vi "ConditioningState-Case.vi"() -> ()   [LabVIEW 2014]
uses:
  ParamsArray.ctl
  Licker.lvclass
  Juicer.lvclass
  Acquisition.lvclass
  Stimulus.lvclass
  state.lvsc/Outputs.ctl
  state.lvsc/Inputs.ctl
  <vilib>/Utility/file.llb/Read From Spreadsheet File (DBL).vi
  state.lvsc
panel:
  out "Waveform Chart":dbl(graph)
  out "size(s) 4":i32
  out "size(s) 3":i32
  out "size(s) 2":i32
  out "size(s)":i32
  out "error out 2":errorcluster
  out "x-y":dbl
  out "Active States":string[](array[string])
  in  "screen_setup":u16(ring) items=["Default", "1"]
  out "queue#":i32
  in  "Probes":enum16{"Testing", "1-5", "6-10"}(ring)=enum."6-10"
  in  "Display":bool
  out "Mon params":dbl[][](array[numeric])=[[100.0, 100.0, 0.0, 0.0], [100.0, 100.0, 100.0, 0.0], [100.0, 100.0, 200.0, 0.0], [100.0, 100.0, 300.0, 0.0], [100.0, 100.0, 400.0, 0.0]]
  out "Air":bool[](array[boolean])
  out "Optical traces":waveform(dbl)[](graph)
  out "CS":bool[](array[boolean])
  out "Number of Licks":dbl[](array[numeric]) caption="#Licks"
  in  "LICK":bool[](array[boolean])=[FALSE, FALSE, FALSE, FALSE, FALSE]
  out "Elapsed Time":dbl[](array[numeric]) caption="Time to Stim"
  out "Rewards Given":dbl[](array[numeric]) caption="#Rew"
  in  "Thr":dbl[](array[numeric])=[10.0, 10.0, 10.0, 10.0, 10.0]
  out "Water":bool[](array[boolean])
  out "Licks":bool[](array[boolean])
  out "error out":errorcluster
  out "Sti":i32
  in  "RUN":bool[](array[boolean])=[FALSE, FALSE, FALSE, FALSE, FALSE]
  out "Lick":i32
  out "Acq":i32
  out "Jui":i32
  in  "REC":bool[](array[boolean])=[FALSE, FALSE, FALSE, FALSE, FALSE]
  in  "Stop":bool
  in  "Params":T1={"Mice ID"=[], "ExpType"=[], "Trial Interval"=[], "Pulse Duration"=[158.0, 152.0, 156.0, 167.0, 172.0], "microL_per_pulse"=[6.0, 6.0, 6.0, 6.0, 6.0], "Response Interval"=[1000.0, 1000.0, 1000.0, 1000.0, 1000.0], "Bad Delay"=[], "Response Period"=[], "liquid_type"="water", "Stimuli"=[], "Rewarded Stimuli"=[], "Air Dur"=400.0} {"Air Dur" format="%#_13g"}
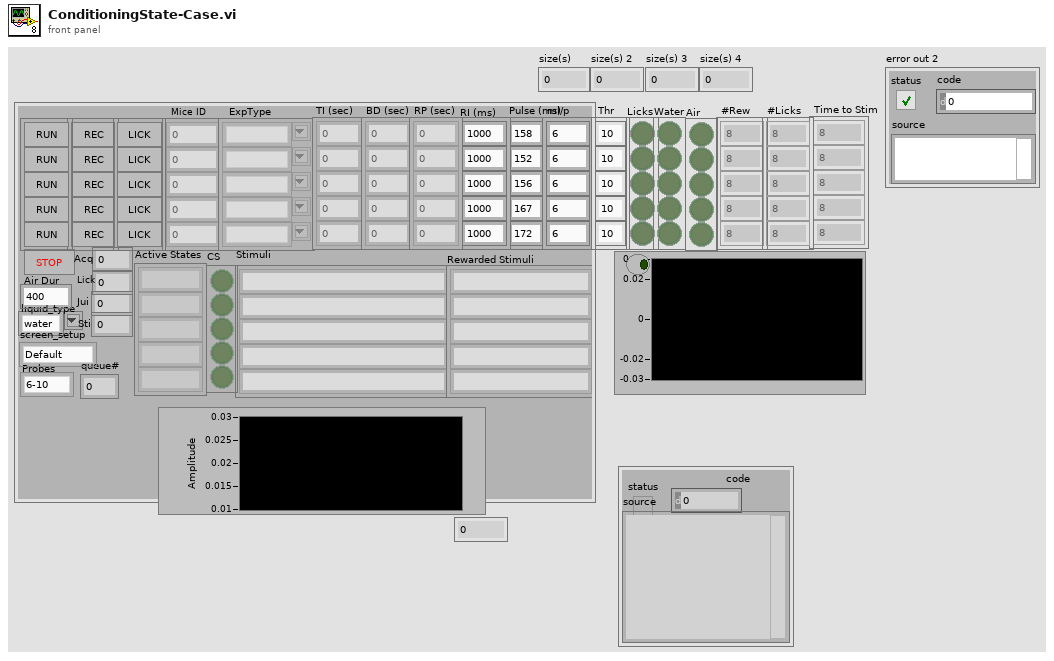
[diagram p1: front panel]
types:
  T1 = typedef "ParamsArray.ctl" = cluster{"Mice ID":dbl[], "ExpType":string[], "Trial Interval":dbl[], "Pulse Duration":dbl[], "microL_per_pulse":dbl[], "Response Interval":dbl[], "Bad Delay":dbl[], "Response Period":dbl[], "liquid_type":string, "Stimuli":string[], "Rewarded Stimuli":string[], "Air Dur":dbl}
  T2 = typedef "state.lvsc/Outputs.ctl" = cluster{"Stimulus.lvclass":refnum<class "Stimulus.lvclass">, "error out":errorcluster, "State":string, "Index":dbl, "Correct Response":bool}
  T3 = enum16{"air_delivery", "beh_session", "stim_periods", "licks", "liquid_delivery", ""}
  T4 = enum16{"Get Time", "Get Elapsed Time", "Reset Elapsed Time"}
  T5 = typedef "state.lvsc/Inputs.ctl" = cluster{"Acquisition.lvclass":refnum<class "Acquisition.lvclass">, "Stimulus.lvclass":refnum<class "Stimulus.lvclass">, "Juicer.lvclass":refnum<class "Juicer.lvclass">, "Index":dbl, "error in (no error)":errorcluster, "Lick":bool, "State":string}
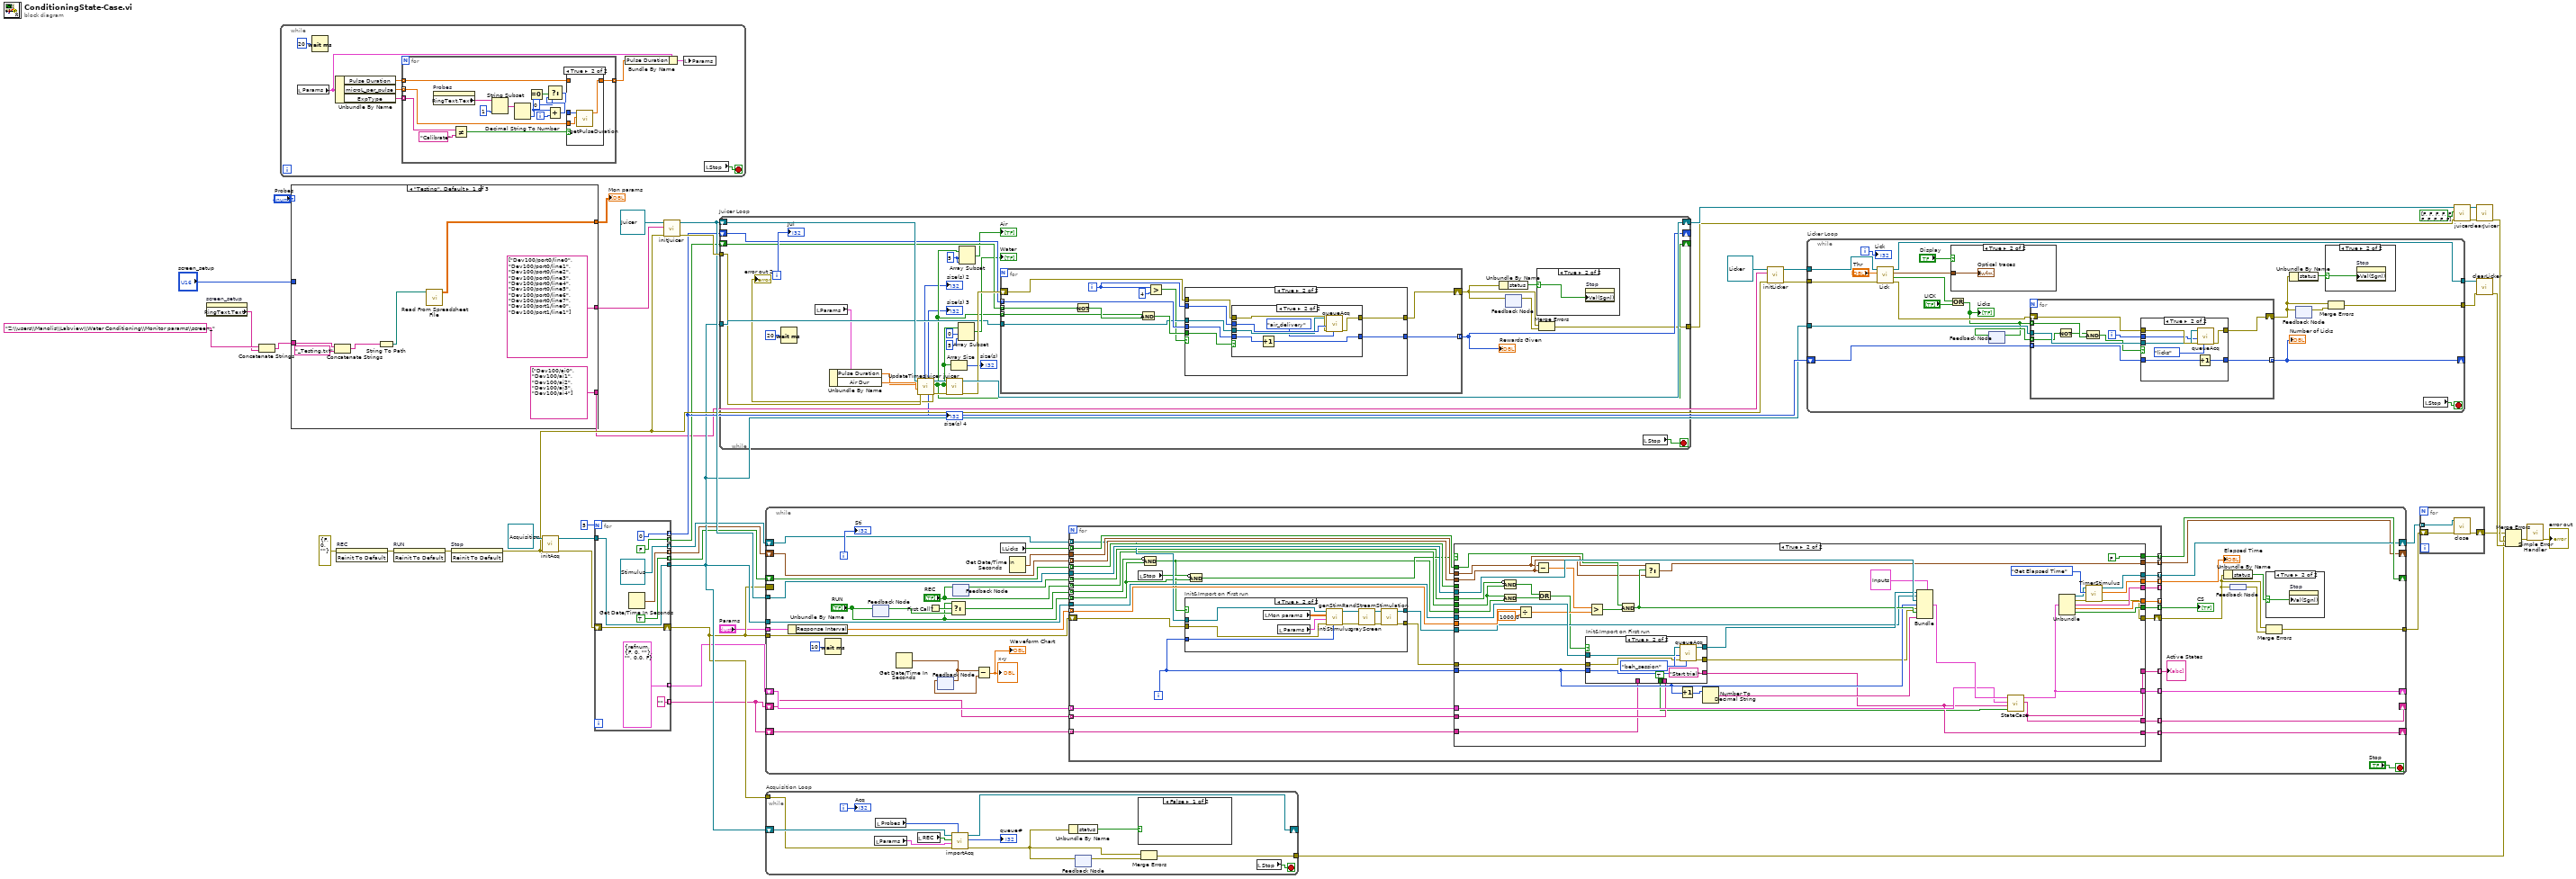
[diagram p0: block diagram]
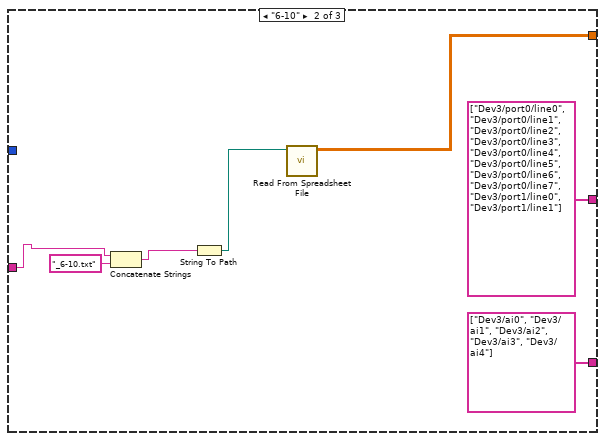
[diagram p3: hidden frame]
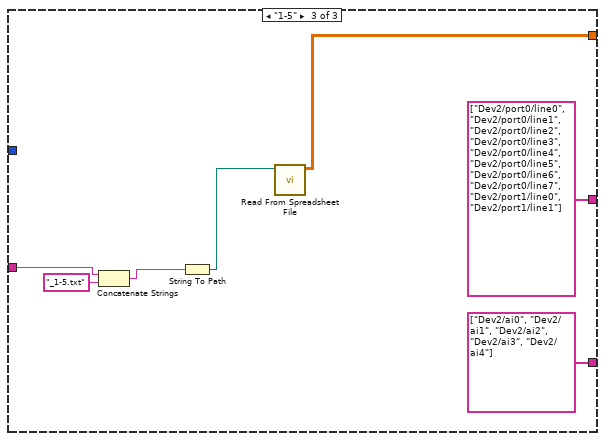
[diagram p4: hidden frame]
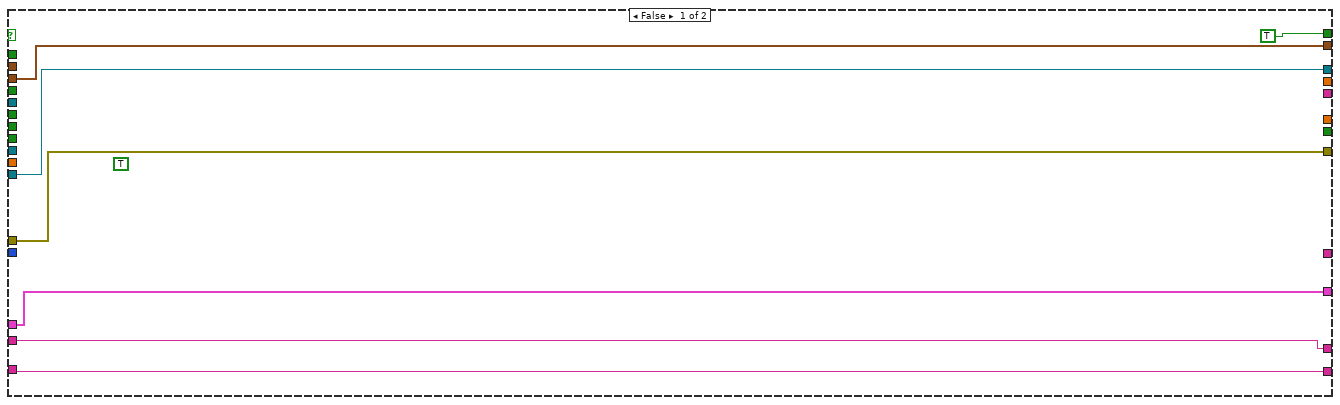
[diagram p7: hidden frame]
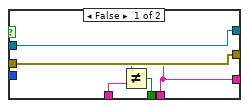
[diagram p8: hidden frame]
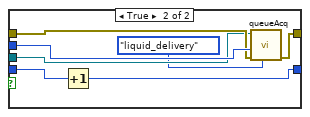
[diagram p14: hidden frame]
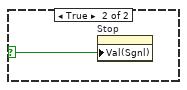
[diagram p16: hidden frame]
diagram:
  n1 = property on="screen_setup" class="Ring (strict)"() -> ("RingText.Text"=w4:string)  [unwired: 2 in, 2 out]
  n2 = Concatenate Strings("Z:\\users\\Manolis\\Labview\\Water Conditioning\\Monitor params\\screen_" ("file path (dialog if empty)"), w4) -> (w3:string)
  n3 = while {
    stop <- w55 stop-if-true
    n4 = local read "Params"() -> (w49:T1)
    n5 = Wait (ms)(milliseconds to wait=u32 20) -> ()  [unwired: 1 out]
    n6 = Unbundle By Name(w49) -> ("Pulse Duration"=w51:dbl[], "microL_per_pulse"=w53:dbl[], "ExpType"=w48:string[])
    n7 = for {
      tunnel: w53 -> [w66] mode=indexing
      tunnel: [w64] -> w52 mode=indexing
      tunnel: w51 -> [w63] mode=indexing
      tunnel: w48 -> [w62] mode=indexing
      i -> [w70]
      n8 = property on="Probes" class="Enum (strict)"() -> ("RingText.Text"=w67:string)  [unwired: 2 in, 2 out]
      n9 = Not Equal?(x=w62, y="Calibrate") -> (x != y?=w61:bool)
      n10 = String Subset(string=w67, length (rest)=1 ("length (rest)")) -> (substring=w69:string)  [unwired: 1 in]
      n11 = Decimal String To Number(string=w69) -> (number=w58:i32)  [unwired: 2 in, 1 out]
      n12 = Equal To 0?(x=w58) -> (x = 0?=w57:bool)
      n13 = Add(x=w58, y=w70) -> (x+y=w60:i32)
      n14 = Select(t=0, s=w57, f=w60) -> (s? t:f=w59:i32)
      n15 = case shown="True" w61 {
        tunnel: w59 -> [_ w74]
        tunnel: w66 -> [_ w73]
        tunnel: [w71 w72] -> w64
        tunnel: w63 -> [w71 _]
        frame False {
        }
        frame True {
          n16 = call "getPulseDuration.vi"("target microL/pulse"=w73, "Probe #"=w74) -> ("Pulse Duration"=w72:dbl)  [unwired: 9 in]
        }
      }
    }
    n17 = Bundle By Name(cluster=w49, "Pulse Duration"=w52) -> (w50:T1)
    n18 = local write "Params"(w50) -> ()
    n19 = local read "Stop"() -> (w55:bool)
  }
  n20 = case shown="\"Testing\", Default" "Probes" {
    tunnel: [w75 w82 w89] -> w16
    tunnel: [string[] ["Dev100/port0/line0", "Dev100/port0/line1", "Dev100/port0/line2", "Dev100/port0/line3", "Dev100/port0/line4", "Dev100/port0/line5", "Dev100/port0/line6", "Dev100/port0/line7", "Dev100/port1/line0", "Dev100/port1/line1"] ("Lines") string[] ["Dev3/port0/line0", "Dev3/port0/line1", "Dev3/port0/line2", "Dev3/port0/line3", "Dev3/port0/line4", "Dev3/port0/line5", "Dev3/port0/line6", "Dev3/port0/line7", "Dev3/port1/line0", "Dev3/port1/line1"] ("Lines") string[] ["Dev2/port0/line0", "Dev2/port0/line1", "Dev2/port0/line2", "Dev2/port0/line3", "Dev2/port0/line4", "Dev2/port0/line5", "Dev2/port0/line6", "Dev2/port0/line7", "Dev2/port1/line0", "Dev2/port1/line1"] ("Lines")] -> w15
    tunnel: [string[] ["Dev100/ai0", "Dev100/ai1", "Dev100/ai2", "Dev100/ai3", "Dev100/ai4"] ("Lines") string[] ["Dev3/ai0", "Dev3/ai1", "Dev3/ai2", "Dev3/ai3", "Dev3/ai4"] ("Lines") string[] ["Dev2/ai0", "Dev2/ai1", "Dev2/ai2", "Dev2/ai3", "Dev2/ai4"] ("Lines")] -> w14
    tunnel: "screen_setup" -> [_ _ _]
    tunnel: w3 -> [w77 w83 w90]
    frame "Testing", Default {
      n21 = Concatenate Strings(w77, "_Testing.txt" ("string")) -> (w78:string)
      n22 = String To Path(string=w78) -> (path=w79:path)
      n23 = call-poly <vilib>:"Read From Spreadsheet File.vi"("file path (dialog if empty)"=w79) -> ("all rows"=w75:dbl[][])  [unwired: 6 in, 4 out]
    }
    frame "6-10" {
      n24 = Concatenate Strings(w83, "_6-10.txt" ("string")) -> (w85:string)
      n25 = String To Path(string=w85) -> (path=w86:path)
      n26 = call-poly <vilib>:"Read From Spreadsheet File.vi"("file path (dialog if empty)"=w86) -> ("all rows"=w82:dbl[][])  [unwired: 6 in, 4 out]
    }
    frame "1-5" {
      n27 = Concatenate Strings(w90, "_1-5.txt" ("string")) -> (w92:string)
      n28 = String To Path(string=w92) -> (path=w93:path)
      n29 = call-poly <vilib>:"Read From Spreadsheet File.vi"("file path (dialog if empty)"=w93) -> ("all rows"=w89:dbl[][])  [unwired: 6 in, 4 out]
    }
  }
  "Mon params" <- w16
  n30 = invoke on="REC" class="Arr (strict)" method="Reinit To Default"(error in=errorcluster {"status"=FALSE, "code"=0, "source"=""} ("error in (no error)")) -> (error out=w33:errorcluster)  [unwired: 2 in, 2 out]
  n31 = invoke on="RUN" class="Arr (strict)" method="Reinit To Default"(error in=w33) -> (error out=w32:errorcluster)  [unwired: 2 in, 2 out]
  n32 = invoke on="Stop" class="Bool (strict)" method="Reinit To Default"(error in=w32) -> (error out=w29:errorcluster)  [unwired: 2 in, 2 out]
  n33 = call-dynamic "initAcq.vi"("error in (no error)"=w29, "Acquisition in"=refnum<class "Acquisition.lvclass"> refnum ("Acquisition.lvclass")) -> ("error out"=w18:errorcluster, "Acquisition out"=w19:refnum<class "Acquisition.lvclass">)  [unwired: 8 in]
  n34 = for {
    N: 5 -> [_]
    tunnel: [refnum<class "Stimulus.lvclass"> refnum ("Stimulus.lvclass")] -> w30 mode=indexing
    shift-right: [w98] -> w23
    shift-left: w18 -> [w98]
    tunnel: [TRUE] -> w22 mode=indexing
    tunnel: [FALSE] -> w21 mode=indexing
    tunnel: [0] -> w25 mode=indexing
    tunnel: [w101] -> w12 mode=indexing
    tunnel: w19 -> [w100]
    tunnel: [w100] -> w24
    tunnel: [T2 {"Stimulus.lvclass"=refnum, "error out"={"status"=FALSE, "code"=0, "source"=""}, "State"="", "Index"=0.0, "Correct Response"=FALSE} ("OutputsOut")] -> w2 mode=indexing
    tunnel: ["" ("StateOut")] -> w1 mode=indexing
    n35 = Get Date/Time In Seconds() -> (seconds since 1Jan1904=w101:timestamp)
  }
  n36 = call-dynamic "initJuicer.vi"("error in (no error)"=w29, "Lines"=w15, "Juicer in"=refnum<class "Juicer.lvclass"> refnum ("Juicer.lvclass")) -> ("error out"=w44:errorcluster, "Juicer out"=w35:refnum<class "Juicer.lvclass">)  [unwired: 7 in]
  n37 = while "Juicer Loop" {
    tunnel: [w116] -> w10
    tunnel: w44 -> [w117]
    shift-right: [w131] -> w11
    shift-left: w35 -> [w132]
    shift-right: [w125] -> _
    shift-left: w25 -> [w126]
    shift-right: [w109] -> _
    shift-left: w21 -> [w124]
    tunnel: w24 -> [w118]
    i -> [w128]
    stop <- w134 stop-if-true
    w120 = 5 ("index")
    n38 = Wait (ms)(milliseconds to wait=u32 20) -> ()  [unwired: 1 out]
    n39 = local read "Params"() -> (w112:T1)
    n40 = Unbundle By Name(w112) -> ("Pulse Duration"=w111:dbl[], "Air Dur"=w113:dbl)
    n41 = call-dynamic "UpdateTimesJuicer.vi"("error in (no error)"=w117, "Air Duration"=w113, "Pulse Duration"=w111, "Juicer in"=w132) -> ("error out"=w110:errorcluster, "Juice"=w109:bool[], "Juicer out"=w133:refnum<class "Juicer.lvclass">, "size(s) 3"=→"size(s) 4":i32, "size(s) 2"=→"size(s) 3":i32, "size(s)"=→"size(s) 2":i32)  [unwired: 2 in]
    "error out 2" <- w110
    n42 = call-dynamic "juicer.vi"("error in (no error)"=w110, "data"=w109, "Juicer in"=w133) -> ("error out"=w130:errorcluster, "Juicer out"=w131:refnum<class "Juicer.lvclass">)  [unwired: 7 in]
    n43 = Array Size(array=w109) -> (size(s)=→"size(s)":i32)
    n44 = Array Subset(array=w109, index=0, length=5) -> (→"Water":bool[])
    n45 = Array Subset(array=w109, index=w120, length=w120) -> (→"Air":bool[])
    n46 = for {
      tunnel: w109 -> [w145] mode=indexing
      shift-right: [w143] -> w115
      shift-left: w130 -> [w144]
      tunnel: w126 -> [w142] mode=indexing
      tunnel: [w141] -> w125 mode=indexing
      tunnel: w124 -> [w140] mode=indexing
      tunnel: w118 -> [w139]
      i -> [w136]
      n47 = Not(x=w140) -> (.not. x?=w146:bool)
      n48 = And(x=w145, y=w146) -> (x .and. y?=w147:bool)
      n49 = Greater?(x=w136, y=4) -> (0:w137:bool)
      n50 = case shown="True" w137 {
        tunnel: w147 -> [w154 w170]
        tunnel: w144 -> [w153 w169]
        tunnel: [w152 w168] -> w143
        tunnel: w142 -> [w151 w167]
        tunnel: [w150 w166] -> w141
        tunnel: w136 -> [w149 w165]
        tunnel: w139 -> [w148 w164]
        frame False {
          n51 = case shown="False" w154 {
            tunnel: w149 -> [_ w163]
            tunnel: w153 -> [w156 w162]
            tunnel: [w156 w161] -> w152
            tunnel: w151 -> [w155 w160]
            tunnel: [w155 w159] -> w150
            tunnel: w148 -> [_ w158]
            frame False {
            }
            frame True {
              n52 = Increment(x=w160) -> (x+1=w159:i32)
              n53 = call-dynamic "queueAcq.vi"("table"=T3."liquid_delivery", "error in (no error)"=w162, "Window Number (0...15)"=w163, "Acquisition in"=w158) -> ("error out"=w161:errorcluster)  [unwired: 5 in, 2 out]
            }
          }
        }
        frame True {
          n54 = case shown="True" w170 {
            tunnel: w165 -> [_ w179]
            tunnel: w169 -> [w172 w178]
            tunnel: [w172 w177] -> w168
            tunnel: w167 -> [w171 w176]
            tunnel: [w171 w175] -> w166
            tunnel: w164 -> [_ w174]
            frame False {
            }
            frame True {
              n55 = Increment(x=w176) -> (x+1=w175:i32)
              n56 = call-dynamic "queueAcq.vi"("table"=T3."air_delivery", "error in (no error)"=w178, "Window Number (0...15)"=w179, "Acquisition in"=w174) -> ("error out"=w177:errorcluster)  [unwired: 5 in, 2 out]
            }
          }
        }
      }
    }
    "Rewards Given" <- w125
    n57 = Unbundle By Name(w115) -> ("status"=w127:bool)
    n58 = feedback #1() -> (w114:errorcluster)  [unwired: 1 in]
    n59 = feedback-in #1(w115) -> ()
    n60 = case shown="True" w127 {
      selector: w127 -> [_ w135]
      frame False {
      }
      frame True {
        n61 = property on="Stop" class="Bool (strict)"("Val(Sgnl)"=w135) -> ()  [unwired: 2 in, 2 out]
      }
    }
    n62 = Merge Errors(w115, w114) -> (w116:errorcluster)
    n63 = local read "Stop"() -> (w134:bool)
    "Jui" <- w128
  }
  n64 = while {
    tunnel: w35 -> [w217]
    shift-right: [w207] -> w28
    shift-left: w30 -> [w191]
    tunnel: w24 -> [w213]
    shift-right: [w212] -> _
    shift-left: w22 -> [w200]
    tunnel: w23 -> [w205]
    tunnel: [w208] -> w27
    border: w23 -> [_]
    shift-right: [w203] -> _
    shift-left: w12 -> [w190]
    tunnel: "Params" -> [w202]
    shift-right: [w188] -> _
    shift-left: w2 -> [w187]
    shift-right: [w186] -> _
    shift-left: w1 -> [w185]
    shift-right: [w184] -> _
    shift-left: w1 -> [w183]
    i -> [w216]
    stop <- "Stop" stop-if-true
    n65 = Unbundle By Name(w202) -> ("Response Interval"=w192:dbl[])
    n66 = Wait (ms)(milliseconds to wait=u32 10) -> ()  [unwired: 1 out]
    n67 = feedback-in #2("RUN") -> ()
    n68 = feedback #2() -> (w198:bool[])  [unwired: 1 in]
    n69 = Get Date/Time In Seconds() -> (seconds since 1Jan1904=w182:timestamp)
    n70 = First Call?() -> (First Call?: T/F=w199:bool)
    n71 = feedback-in #3(w182) -> ()
    n72 = feedback #3() -> (w181:timestamp)  [unwired: 1 in]
    n73 = Select(t="RUN", s=w199, f=w198) -> (s? t:f=w194:bool[])
    n74 = feedback #4() -> (w196:bool[])  [unwired: 1 in]
    n75 = feedback-in #4("REC") -> ()
    n76 = Subtract(x=w182, y=w181) -> (x-y=→"x-y" →"Waveform Chart":dbl)
    n77 = local read "Licks"() -> (w197:bool[])
    n78 = Get Date/Time In Seconds() -> (seconds since 1Jan1904=w204:timestamp)
    n79 = for {
      tunnel: "RUN" -> [w229] mode=indexing
      tunnel: w217 -> [w252]
      shift-right: [w251] -> w210
      shift-left: w205 -> [w237]
      tunnel: w213 -> [w242]
      tunnel: w200 -> [w250] mode=indexing
      tunnel: [w249] -> w212 mode=indexing
      tunnel: [w248] -> w211 mode=indexing
      tunnel: [w247] -> _ mode=indexing
      tunnel: [w246] -> _ mode=indexing
      tunnel: w191 -> [w235] mode=indexing
      tunnel: [w245] -> w207 mode=indexing
      tunnel: [w244] -> w206 mode=indexing
      tunnel: w197 -> [w243] mode=indexing
      tunnel: "REC" -> [w233] mode=indexing
      tunnel: w190 -> [w240] mode=indexing
      tunnel: w204 -> [w241]
      tunnel: [w239] -> w203 mode=indexing
      tunnel: w192 -> [w238] mode=indexing
      tunnel: w194 -> [w231] mode=indexing
      tunnel: w196 -> [w227] mode=indexing
      tunnel: [w225] -> w189 mode=indexing
      tunnel: [w224] -> w188 mode=indexing
      tunnel: w187 -> [w223] mode=indexing
      tunnel: [w222] -> w186 mode=indexing
      tunnel: w185 -> [w221] mode=indexing
      tunnel: [w220] -> w184 mode=indexing
      tunnel: w183 -> [w219] mode=indexing
      i -> [w232]
      n80 = local read "Stop"() -> (w230:bool)
      n81 = Compound Arithmetic op=AND(invert w231, w229) -> (w226:bool)
      n82 = case "Init&Import on First run" shown="True" w226 {
        tunnel: [w254 w256] -> w236
        tunnel: w237 -> [w254 w260]
        tunnel: w232 -> [_ w259]
        tunnel: [w253 w261] -> w234
        tunnel: w235 -> [w253 w255]
        frame False {
        }
        frame True {
          n83 = local read "Mon params"() -> (w257:dbl[][])
          n84 = local read "Params"() -> (w258:T1)
          n85 = call-dynamic "intiStimulus.vi"("index"=w259, "error in (no error)"=w260, "Params"=w258, "Monitor parameters"=w257, "Stimulus in"=w255) -> ("error out"=w263:errorcluster, "Stimulus out"=w262:refnum<class "Stimulus.lvclass">)  [unwired: 5 in]
          n86 = call-dynamic "grayScreen.vi"("error in (no error)"=w263, "Stimulus in"=w262) -> ("error out"=w265:errorcluster, "Stimulus out"=w264:refnum<class "Stimulus.lvclass">)  [unwired: 8 in]
          n87 = call-dynamic "genStimRandStreamStimulation.vi"("error in (no error)"=w265, "Stimulus in"=w264) -> ("error out"=w256:errorcluster, "Stimulus out"=w261:refnum<class "Stimulus.lvclass">)  [unwired: 8 in]
        }
      }
      n88 = Compound Arithmetic op=AND(invert w230, w229) -> (w228:bool)
      n89 = case shown="True" w228 {
        tunnel: w242 -> [_ w306]
        tunnel: w234 -> [w272 w290]
        tunnel: w252 -> [_ w316]
        tunnel: [w271 w283] -> w251
        tunnel: [w272 w292] -> w245
        tunnel: w236 -> [w271 w304]
        tunnel: w232 -> [_ w293]
        tunnel: w250 -> [_ _]
        tunnel: [TRUE FALSE] -> w249
        tunnel: [_ w314] -> w248
        tunnel: [_ w310] -> w247
        tunnel: [_ w309] -> w246
        tunnel: [_ w291] -> w244
        tunnel: w243 -> [_ w299]
        tunnel: w241 -> [_ w295]
        tunnel: w240 -> [w269 w296]
        tunnel: [w269 w294] -> w239
        tunnel: w238 -> [_ w298]
        tunnel: w233 -> [_ w286]
        tunnel: w227 -> [_ w289]
        tunnel: w226 -> [_ w285]
        tunnel: [_ w277] -> w225
        tunnel: [w268 w279] -> w224
        tunnel: w223 -> [w268 w278]
        tunnel: [w267 w277] -> w222
        tunnel: w221 -> [w267 w276]
        tunnel: [w266 w275] -> w220
        tunnel: w219 -> [w266 w274]
        frame False {
          (unwired) TRUE
        }
        frame True {
          n90 = And(x=w286, y=w285) -> (x .and. y?=w287:bool)
          n91 = Compound Arithmetic op=AND(invert w289, w286) -> (w288:bool)
          n92 = Divide(x=w298, y=1000.0) -> (x/y=w303:dbl)
          n93 = Subtract(x=w295, y=w296) -> (x-y=w300:dbl)
          n94 = Or(x=w288, y=w287) -> (x .or. y?=w284:bool)
          n95 = case "Init&Import on First run" shown="True" w284 {
            tunnel: [w320 w329] -> w305
            tunnel: [w321 w328] -> w281
            tunnel: w306 -> [w320 w327]
            tunnel: w304 -> [w321 w324]
            tunnel: w293 -> [_ w325]
            tunnel: w276 -> [w318 _]
            tunnel: [w318 "Start trial" ("StateOut")] -> w275
            tunnel: w274 -> [w319 _]
            tunnel: [w317 TRUE] -> w273
            frame False {
              n96 = Not Equal?(x=w318, y=w319) -> (x != y?=w317:bool)
            }
            frame True {
              n97 = call-dynamic "queueAcq.vi"("table"=T3."beh_session", "error in (no error)"=w324, "Window Number (0...15)"=w325, "Acquisition in"=w327) -> ("error out"=w328:errorcluster, "Acquisition out"=w329:refnum<class "Acquisition.lvclass">)  [unwired: 5 in, 1 out]
            }
          }
          n98 = Greater?(x=w300, y=w303) -> (0:w301:bool)
          n99 = And(x=w299, y=w301) -> (x .and. y?=w297:bool)
          n100 = Select(t=w295, s=w297, f=w296) -> (s? t:f=w294:timestamp)
          n101 = Increment(x=w293) -> (x+1=w312:i32)
          n102 = Number To Decimal String(number=w312) -> (decimal integer string=w282:string)  [unwired: 1 in]
          n103 = Bundle(cluster=T5 {"Acquisition.lvclass"=refnum, "Stimulus.lvclass"=refnum, "Juicer.lvclass"=refnum, "Index"=0.0, "error in (no error)"={"status"=FALSE, "code"=0, "source"=""}, "Lick"=FALSE, "State"=""} ("Inputs"), "Acquisition.lvclass"=w305, "Stimulus.lvclass"=w290, "Juicer.lvclass"=w316, "Index"=w293, "error in (no error)"=w281, "Lick"=w297, "State"=w282) -> (w280:T5)
          n104 = call "StateCase.vi"("Same State?"=w273, "StateIn"=w275, "OutputsIn"=w278, "Inputs"=w280) -> ("StateOut"=w277:string, "OutputsOut"=w279:T2)  [unwired: 6 in]
          n105 = Unbundle(w279) -> ("Stimulus.lvclass"=w308:refnum<class "Stimulus.lvclass">, "error out"=w307:errorcluster, "State"=w310:string, "Index"=w309:dbl, "Correct Response"=w291:bool)
          n106 = call-dynamic "TimerStimulus.vi"("error in (no error)"=w307, "Method"=T4."Get Elapsed Time", "Stimulus in"=w308) -> ("error out"=w283:errorcluster, "Time"=w314:dbl, "Stimulus out"=w292:refnum<class "Stimulus.lvclass">)  [unwired: 5 in, 1 out]
        }
      }
    }
    "Elapsed Time" <- w211
    "CS" <- w206
    "Active States" <- w189
    n107 = Unbundle By Name(w210) -> ("status"=w214:bool)
    n108 = feedback-in #5(w210) -> ()
    n109 = feedback #5() -> (w209:errorcluster)
    n110 = case shown="True" w214 {
      selector: w214 -> [_ w218]
      frame False {
      }
      frame True {
        n111 = property on="Stop" class="Bool (strict)"("Val(Sgnl)"=w218) -> ()  [unwired: 2 in, 2 out]
      }
    }
    n112 = Merge Errors(w210, w209) -> (w208:errorcluster)
    "Sti" <- w216
  }
  n113 = while "Acquisition Loop" {
    tunnel: w23 -> [w339]
    tunnel: [w334] -> w37
    shift-right: [w341] -> _
    shift-left: w24 -> [w340]
    i -> [w342]
    stop <- w333 stop-if-true
    n114 = local read "Params"() -> (w337:T1)
    n115 = local read "Probes"() -> (w330:enum16{"Testing", "1-5", "6-10"})
    n116 = local read "REC"() -> (w332:bool[])
    n117 = call-dynamic "importAcq.vi"("Probes"=w330, "error in (no error)"=w339, "Params"=w337, "REC"=w332, "Acquisition in"=w340) -> ("error out"=w335:errorcluster, "# elements in queue"=→"queue#":i32, "Acquisition out"=w341:refnum<class "Acquisition.lvclass">)  [unwired: 4 in]
    n118 = Unbundle By Name(w335) -> ("status"=w338:bool)
    n119 = feedback #6() -> (w336:errorcluster)  [unwired: 1 in]
    n120 = feedback-in #6(w335) -> ()
    n121 = case shown="False" w338 {
      selector: w338 -> [_ w343]
      frame False {
      }
      frame True {
        n122 = property on="Stop" class="Bool (strict)"("Val(Sgnl)"=w343) -> ()  [unwired: 2 in, 2 out]
      }
    }
    n123 = Merge Errors(w335, w336) -> (w334:errorcluster)
    n124 = local read "Stop"() -> (w333:bool)
    "Acq" <- w342
  }
  n125 = call-dynamic "initLicker.vi"("error in (no error)"=w29, "Lines"=w14, "Licker in"=refnum<class "Licker.lvclass"> refnum ("Licker.lvclass")) -> ("error out"=w42:errorcluster, "Licker out"=w45:refnum<class "Licker.lvclass">)  [unwired: 7 in]
  n126 = while "Licker Loop" {
    tunnel: w42 -> [w360]
    tunnel: [w346] -> w40
    tunnel: w45 -> [w362]
    tunnel: [w361] -> w43
    shift-right: [w350] -> _
    shift-left: w25 -> [w351]
    tunnel: w24 -> [w353]
    i -> [w356]
    stop <- w363 stop-if-true
    n127 = call-dynamic "Lick.vi"("error in (no error)"=w360, "% decrease Thr"="Thr", "Licker in"=w362) -> ("error out"=w357:errorcluster, "Lick?"=w354:bool[], "data"=w359:waveform(dbl)[], "Licker out"=w361:refnum<class "Licker.lvclass">)  [unwired: 5 in]
    n128 = Or(x=w354, y="LICK") -> (x .or. y?=w344:bool[])
    "Licks" <- w344
    n129 = case shown="True" "Display" {
      tunnel: w359 -> [_ w364]
      frame False {
      }
      frame True {
        "Optical traces" <- w364
      }
    }
    n130 = feedback-in #7(w344) -> ()
    n131 = feedback #7() -> (w352:bool[])  [unwired: 1 in]
    n132 = for {
      tunnel: w344 -> [w371] mode=indexing
      shift-right: [w374] -> w347
      shift-left: w357 -> [w375]
      tunnel: w352 -> [w370] mode=indexing
      tunnel: w351 -> [w367] mode=indexing
      tunnel: [w366] -> w350 mode=indexing
      tunnel: w353 -> [w373]
      i -> [w372]
      n133 = Not(x=w370) -> (.not. x?=w369:bool)
      n134 = And(x=w369, y=w371) -> (x .and. y?=w368:bool)
      n135 = case shown="True" w368 {
        tunnel: w372 -> [_ w381]
        tunnel: w375 -> [w377 w384]
        tunnel: [w377 w383] -> w374
        tunnel: w373 -> [_ w382]
        tunnel: w367 -> [w376 w380]
        tunnel: [w376 w379] -> w366
        frame False {
        }
        frame True {
          n136 = Increment(x=w380) -> (x+1=w379:i32)
          n137 = call-dynamic "queueAcq.vi"("table"=T3."licks", "error in (no error)"=w384, "Window Number (0...15)"=w381, "Acquisition in"=w382) -> ("error out"=w383:errorcluster)  [unwired: 5 in, 2 out]
        }
      }
    }
    "Number of Licks" <- w350
    n138 = Unbundle By Name(w347) -> ("status"=w355:bool)
    n139 = feedback #8() -> (w348:errorcluster)  [unwired: 1 in]
    n140 = feedback-in #8(w347) -> ()
    n141 = case shown="True" w355 {
      selector: w355 -> [_ w365]
      frame False {
      }
      frame True {
        n142 = property on="Stop" class="Bool (strict)"("Val(Sgnl)"=w365) -> ()  [unwired: 2 in, 2 out]
      }
    }
    n143 = Merge Errors(w347, w348) -> (w346:errorcluster)
    n144 = local read "Stop"() -> (w363:bool)
    "Lick" <- w356
  }
  n145 = for {
    tunnel: w28 -> [w387] mode=indexing
    shift-right: [w385] -> w26
    shift-left: w27 -> [w386]
    n146 = call-dynamic "close.vi"("error in (no error)"=w386, "Stimulus in"=w387) -> ("error out"=w385:errorcluster)  [unwired: 8 in, 1 out]
  }
  n147 = call-dynamic "juicer.vi"("error in (no error)"=w10, "data"=bool[] [FALSE, FALSE, FALSE, FALSE, FALSE, FALSE, FALSE, FALSE, FALSE, FALSE], "Juicer in"=w11) -> ("error out"=w9:errorcluster, "Juicer out"=w8:refnum<class "Juicer.lvclass">)  [unwired: 7 in]
  n148 = call-dynamic "clearJuicer.vi"("error in (no error)"=w9, "Juicer in"=w8) -> ("error out"=w38:errorcluster)  [unwired: 8 in, 1 out]
  n149 = call-dynamic "clearLicker.vi"("error in (no error)"=w40, "Licker in"=w43) -> ("error out"=w39:errorcluster)  [unwired: 8 in, 1 out]
  n150 = Merge Errors(w26, w37, w38, w39) -> (w36:errorcluster)
  n151 = call <vilib>:"Simple Error Handler.vi"("error in (no error)"=w36) -> ("error out"=→"error out":errorcluster)  [unwired: 4 in, 4 out]
